vi "LinearQuadraticRegulator_New_SystemELMS.vi"(6 "dt_Seconds":dbl=0.02, 8 "Relms":T2, 9 "Qelms":T2, 11 "LINEARSYSTEM":T1) -> (0 "Error":bool, 3 "LinearQuadraticRegulator":T3)   [LabVIEW 2019, in "Trajectory_Library.lvlib"]
doc: "Contains the controller coefficients and logic for a linear-quadratic regulator (LQR). LQRs use\nthe control law u = K(r - x).\n \nFor more on the underlying math, read\nhttps://file.tavsys.net/control/controls-engineering-in-frc.pdf.\n\nConstructs a controller with the given coefficients and plant. Rho is defaulted to 1.\n\nInputs:\n - LinearSystem - The plant being controlled.\n - qelms -- The maximum desired error tolerance for each state.\n - relms -- The maximum desired control effort for each input.\n - dtSeconds -- Discretization timestep.\n\nOutputs:\n - LinearQuadraticRegullator -- controller data cluster\n - Error -- If TRUE, and error occured."
uses:
  Trajectory_Library.lvlib
  <vilib>/Analysis/Matrix/Datatypes/RealMatrix.ctl
  <vilib>/Analysis/Matrix/NI_Matrix.lvlib
  TypeDef/LINEAR_QUADRATIC_REGULATOR.ctl
  TypeDef/LINEAR_SYSTEM.ctl
panel:
  # "<States,1>"
  # "<Inputs,1>"
  # "<States,States>"
  # "<States,Inputs>"
  # "<Outputs,States>"
  # "<Outputs,Inputs>"
  # "Ref State <States,1>"
  # "Comp and capped \noutput <Inputs,1>"
  # "Controller gain\n<Inputs,States>"
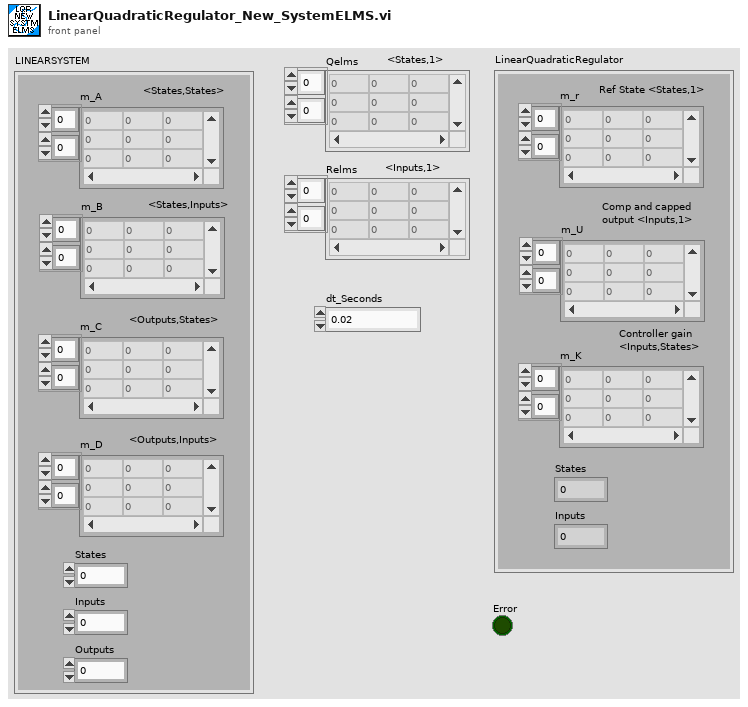
[diagram p1: front panel]
types:
  T1 = typedef "Trajectory_Library.lvlib/LINEAR_SYSTEM.ctl" = cluster{"m_A":T2, "m_B":T2, "m_C":T2, "m_D":T2, "States":i32, "Inputs":i32, "Outputs":i32}
  T2 = typedef "NI_Matrix.lvlib/RealMatrix.ctl" = dbl[][]
  T3 = typedef "Trajectory_Library.lvlib/LINEAR_QUADRATIC_REGULATOR.ctl" = cluster{"m_r":T2, "m_U":T2, "m_K":T2, "States":i32, "Inputs":i32}
  T4 = typedef "WPILib_Math.lvlib/LINEAR_QUADRATIC_REGULATOR.ctl" = cluster{"m_r":T2, "m_U":T2, "m_K":T2, "States":i32, "Inputs":i32}
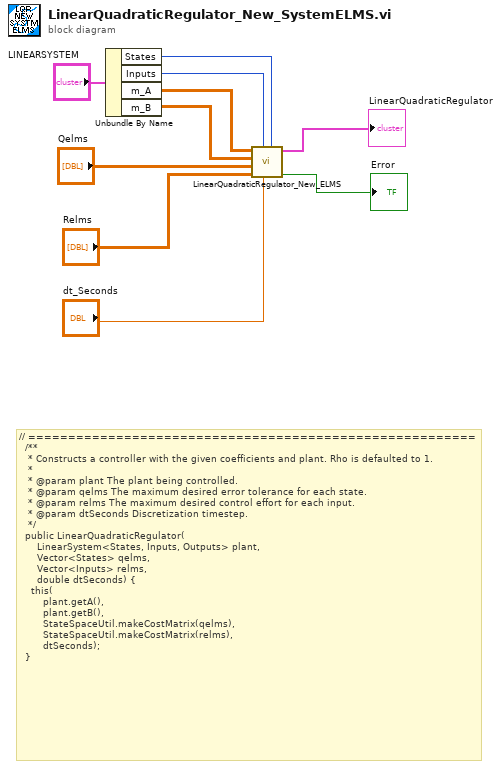
[diagram p0: block diagram]
diagram:
  # "// ========================================================\n  /**\n   * Constructs a controller with the given coefficients and plant. Rho is defaulted to 1.\n   *\n   * @param plant The plant being controlled.\n   * @param qelms The maximum desired error tolerance for each state.\n   * @param relms The maximum desired control effort for each input.\n   * @param dtSeconds Discretization timestep.\n   */\n  public LinearQuadraticRegulator(\n      LinearSystem<States, Inputs, Outputs> plant,\n      Vector<States> qelms,\n      Vector<Inputs> relms,\n      double dtSeconds) {\n    this(\n        plant.getA(),\n        plant.getB(),\n        StateSpaceUtil.makeCostMatrix(qelms),\n        StateSpaceUtil.makeCostMatrix(relms),\n        dtSeconds);\n  }"
  n1 = Unbundle By Name("LINEARSYSTEM") -> ("States"=w9:i32, "Inputs"=w8:i32, "m_A"=w7:T2, "m_B"=w6:T2)
  n2 = call "LinearQuadraticRegulator_New_ELMS.vi"("States"=w9, "dt_Seconds"="dt_Seconds", "Inputs"=w8, "Relms"="Relms", "Qelms"="Qelms", "B"=w6, "A"=w7) -> ("Error"=→"Error":bool, "LinearQuadraticRegulator"=→"LinearQuadraticRegulator":T4)  [unwired: 3 in]
